vi "get_key_type.vi"(8 "error in (no error)":errorcluster, 10 "item_name":string, 11 "Table in":refnum<class "Table.lvclass">) -> (0 "error out":errorcluster, 1 "value_type":string, 2 "item_type":string, 3 "Table out":refnum<class "Table.lvclass">)   [LabVIEW 2020]
uses:
  Table.lvclass/Table.ctl
  dragon_toml_64.dll
  toml_edit.lvlib
  Table.lvclass
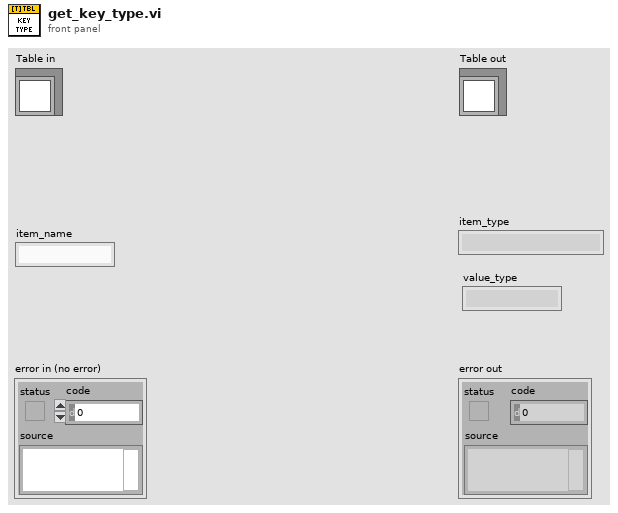
[diagram p1: front panel]
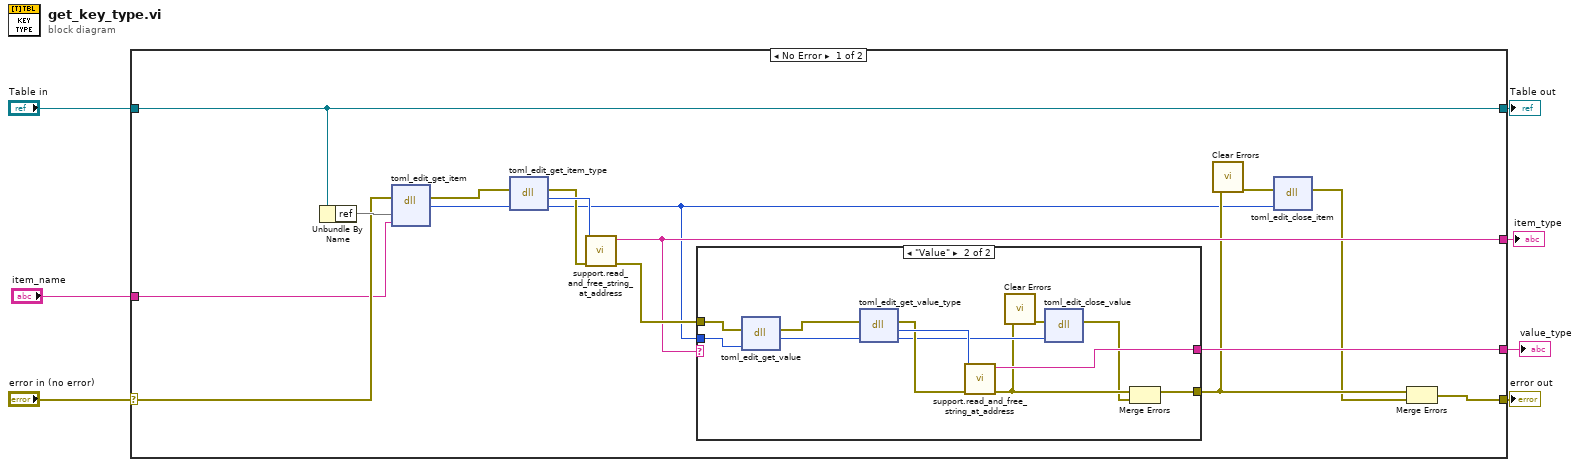
[diagram p0: block diagram]
diagram:
  n1 = case shown="No Error" "error in (no error)" {
    selector: "error in (no error)" -> [w21 w38]
    tunnel: [w15 w38] -> w6
    tunnel: [w22 w37] -> w4
    tunnel: "Table in" -> [w22 w37]
    tunnel: [w12 _] -> w3
    tunnel: "item_name" -> [w20 _]
    tunnel: [w13 _] -> w1
    frame No Error {
      n2 = Unbundle By Name(w22) -> ("ref"=w23)
      n3 = dll-call lib="C:/Projects/labview-project-load-tools/rust_src/toml_edit_dll/lv_src/dragon_toml_*.dll" fn="toml_edit_get_item"(error in=w21, "table"=w23, "item_name"=w20) -> (error out=w18:errorcluster, "item"=w19:u64)  [unwired: 4 in, 1 out]
      n4 = dll-call lib="C:/Projects/labview-project-load-tools/rust_src/toml_edit_dll/lv_src/dragon_toml_*.dll" fn="toml_edit_get_item_type"(error in=w18, "item"=w19) -> (error out=w16:errorcluster, "string_ptr"=w17:u64, "item"=w8:u64)  [unwired: 2 in, 1 out]
      n5 = call "support.read_and_free_string_at_address.vi"("error in (no error)"=w16, "string_ptr"=w17) -> ("error out"=w14:errorcluster, "string"=w12:string)  [unwired: 8 in]
      n6 = case shown="\"Value\"" w12 {
        tunnel: w8 -> [_ w32]
        tunnel: w14 -> [w24 w31]
        tunnel: [w24 w26] -> w11
        tunnel: [_ w34] -> w13
        frame Default {
        }
        frame "Value" {
          n7 = dll-call lib="C:/Projects/labview-project-load-tools/rust_src/toml_edit_dll/lv_src/dragon_toml_*.dll" fn="toml_edit_get_value"(error in=w31, "item"=w32) -> (error out=w30:errorcluster, "value"=w33:u64)  [unwired: 3 in, 1 out]
          n8 = dll-call lib="C:/Projects/labview-project-load-tools/rust_src/toml_edit_dll/lv_src/dragon_toml_*.dll" fn="toml_edit_get_value_type"(error in=w30, "item"=w33) -> (error out=w35:errorcluster, "string_ptr"=w36:u64, "item"=w29:u64)  [unwired: 2 in, 1 out]
          n9 = call "support.read_and_free_string_at_address.vi"("error in (no error)"=w35, "string_ptr"=w36) -> ("error out"=w27:errorcluster, "string"=w34:string)  [unwired: 8 in]
          n10 = call <vilib>:"Clear Errors.vi"("error in (no error)"=w27) -> ("error out"=w28:errorcluster)  [unwired: 5 in, 1 out]
          n11 = dll-call lib="C:/Projects/labview-project-load-tools/rust_src/toml_edit_dll/lv_src/dragon_toml_*.dll" fn="toml_edit_close_value"(error in=w28, "value"=w29) -> (error out=w25:errorcluster)  [unwired: 4 in, 1 out]
          n12 = Merge Errors(w27, w25) -> (w26:errorcluster)
        }
      }
      n13 = call <vilib>:"Clear Errors.vi"("error in (no error)"=w11) -> ("error out"=w10:errorcluster)  [unwired: 5 in, 1 out]
      n14 = dll-call lib="C:/Projects/labview-project-load-tools/rust_src/toml_edit_dll/lv_src/dragon_toml_*.dll" fn="toml_edit_close_item"(error in=w10, "item"=w8) -> (error out=w9:errorcluster)  [unwired: 4 in, 1 out]
      n15 = Merge Errors(w11, w9) -> (w15:errorcluster)
    }
    frame Error {
    }
  }
  "error out" <- w6
  "Table out" <- w4
  "item_type" <- w3
  "value_type" <- w1
